vi "Get KPRO Output  Indices.vi"(0 "KPRO Culmulative \ntest report header 2":T1=["Measurement Time", "Current Absolute Depth (Uncorrected)", "Corrected Depth", "Depth Rate", "Flow", "Feet of Stainless Steel Used", "In line Pressure Sensor", "IK", "Corrected Headloss", "Atmospheric Pressure (global)", "Depth to Water Table (global)", "Height of Box (global)", "Resevoir Pressure (global)", "Seconds since Jan 1 1904", "Marker", "Downhole Pressure Sensor (ft/H20)", "Downhole Pressure Sensor (V)", "DHT Depth to Water", "DHT IK", "Current Relative Depth", "Previous Relative Depth"]) -> (1 "Height of Box (global)":i32, 2 "Feet of Stainless Steel":i32, 3 "Depth Rate Index":i32, 4 "Measurement Time Index":i32, 5 "Depth to Water Table (global)":i32, 6 "Uncorrected Depth Index":i32, 8 "Headloss index":i32, 10 "Corrected Depth Index":i32, 12 "Flow Index":i32, 13 "Pressure Index":i32, 14 "IK index":i32)   [LabVIEW 2016]
uses:
  controls/KPro Header Control 1.ctl
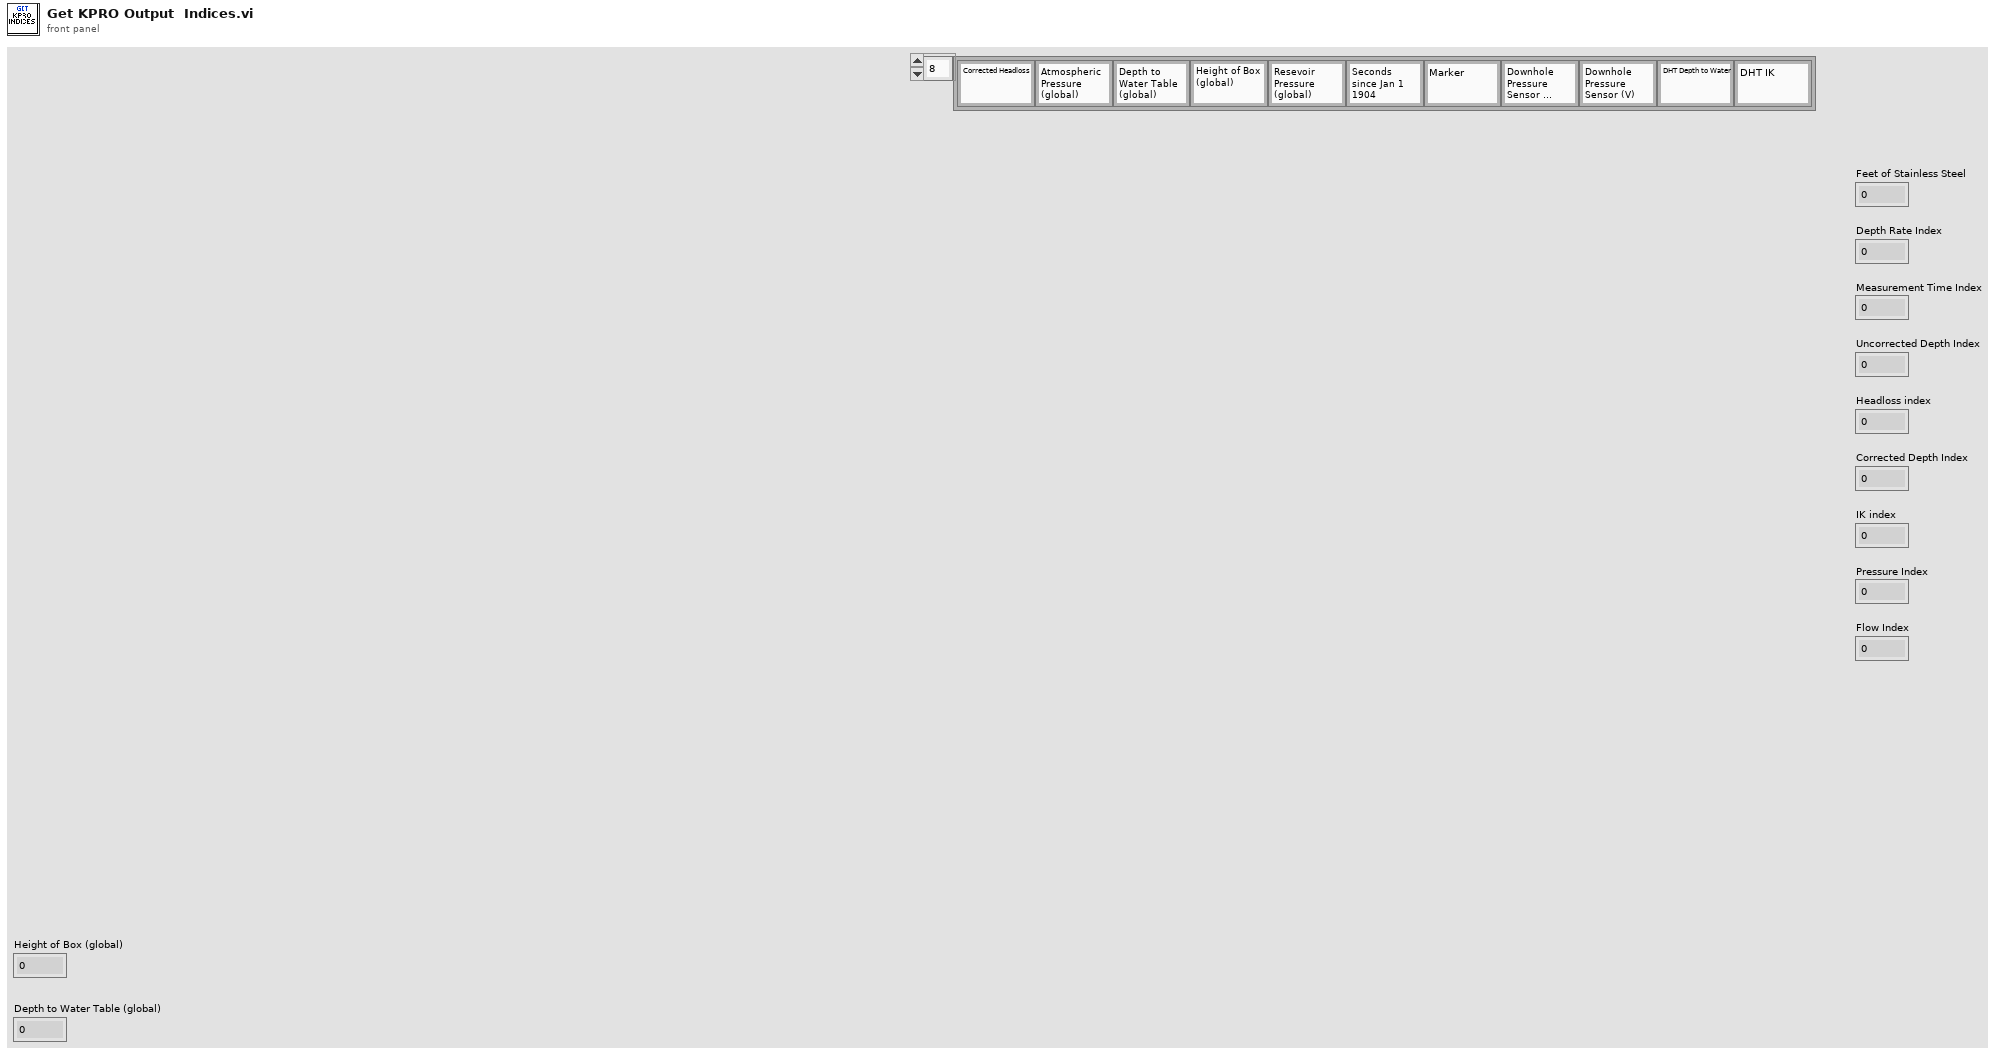
[diagram p1: front panel]
types:
  T1 = typedef "KPro Header Control 1.ctl" = string[]
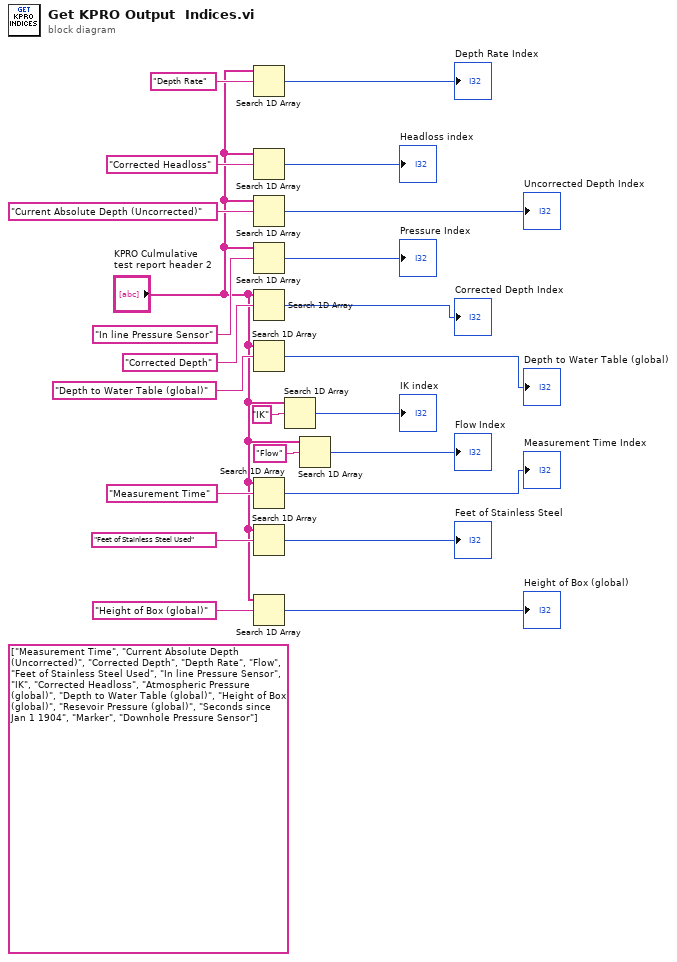
[diagram p0: block diagram]
diagram:
  (unwired) string[] ["Measurement Time", "Current Absolute Depth (Uncorrected)", "Corrected Depth", "Depth Rate", "Flow", "Feet of Stainless Steel Used", "In line Pressure Sensor", "IK", "Corrected Headloss", "Atmospheric Pressure (global)", "Depth to Water Table (global)", "Height of Box (global)", "Resevoir Pressure (global)", "Seconds since Jan 1 1904", "Marker", "Downhole Pressure Sensor"] ("Array")
  n1 = Search 1D Array(1D array="KPRO Culmulative \ntest report header 2", element="Depth Rate") -> (index of element=→"Depth Rate Index":i32)  [unwired: 1 in]
  n2 = Search 1D Array(1D array="KPRO Culmulative \ntest report header 2", element="Corrected Headloss") -> (index of element=→"Headloss index":i32)  [unwired: 1 in]
  n3 = Search 1D Array(1D array="KPRO Culmulative \ntest report header 2", element="Current Absolute Depth (Uncorrected)") -> (index of element=→"Uncorrected Depth Index":i32)  [unwired: 1 in]
  n4 = Search 1D Array(1D array="KPRO Culmulative \ntest report header 2", element="In line Pressure Sensor") -> (index of element=→"Pressure Index":i32)  [unwired: 1 in]
  n5 = Search 1D Array(1D array="KPRO Culmulative \ntest report header 2", element="Corrected Depth") -> (index of element=→"Corrected Depth Index":i32)  [unwired: 1 in]
  n6 = Search 1D Array(1D array="KPRO Culmulative \ntest report header 2", element="Depth to Water Table (global)") -> (index of element=→"Depth to Water Table (global)":i32)  [unwired: 1 in]
  n7 = Search 1D Array(1D array="KPRO Culmulative \ntest report header 2", element="Measurement Time") -> (index of element=→"Measurement Time Index":i32)  [unwired: 1 in]
  n8 = Search 1D Array(1D array="KPRO Culmulative \ntest report header 2", element="Feet of Stainless Steel Used") -> (index of element=→"Feet of Stainless Steel":i32)  [unwired: 1 in]
  n9 = Search 1D Array(1D array="KPRO Culmulative \ntest report header 2", element="Height of Box (global)") -> (index of element=→"Height of Box (global)":i32)  [unwired: 1 in]
  n10 = Search 1D Array(1D array="KPRO Culmulative \ntest report header 2", element="IK") -> (index of element=→"IK index":i32)  [unwired: 1 in]
  n11 = Search 1D Array(1D array="KPRO Culmulative \ntest report header 2", element="Flow") -> (index of element=→"Flow Index":i32)  [unwired: 1 in]
